vi "Create All Message Queues.vi"(8 "error in (no error)":errorcluster) -> (0 "error out":errorcluster, 3 "Message Queues out":T1)   [LabVIEW 2026, in "Temp Monitor Message Queue.lvlib"]
doc: "This VI creates and initializes all the message queues for the Temperature Monitoring application."
uses:
  Temp Monitor Message Queue.lvlib
  All Message Queues.ctl
  Message Cluster.ctl
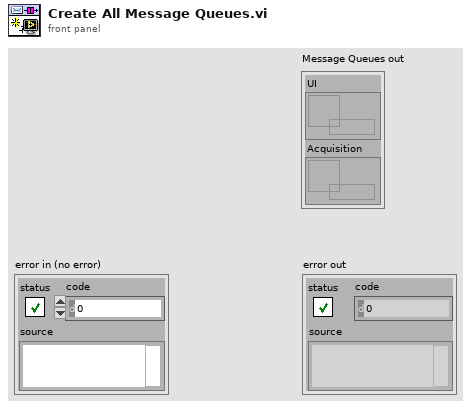
[diagram p1: front panel]
types:
  T1 = typedef "Temp Monitor Message Queue.lvlib/All Message Queues.ctl" = cluster{"UI":refnum<queue>, "Acquisition":refnum<queue>}
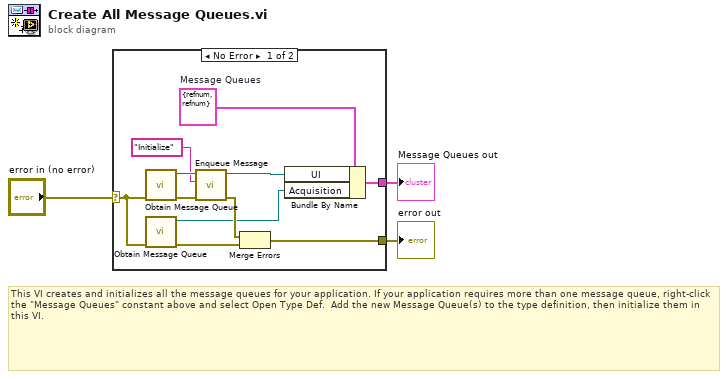
[diagram p0: block diagram]
diagram:
  # "This VI creates and initializes all the message queues for your application. If your application requires more than one message queue, right-click the \"Message Queues\" constant above and select Open Type Def.  Add the new Message Queue(s) to the type definition, then initialize them in this VI."
  n1 = case shown="No Error" "error in (no error)" {
    selector: "error in (no error)" -> [w9 w15]
    tunnel: [w6 w15] -> w3
    tunnel: [w12 _] -> w2
    frame No Error {
      w13 = T1 {"UI"=refnum, "Acquisition"=refnum}  # Message Queues
      n2 = call "Obtain Message Queue.vi"("error in (no error)"=w9) -> ("error out"=w11:errorcluster, "Message Queue"=w10:refnum<queue>)  [unwired: 9 in]
      n3 = call "Obtain Message Queue.vi"("error in (no error)"=w9) -> ("error out"=w4:errorcluster, "Message Queue"=w5:refnum<queue>)  [unwired: 9 in]
      n4 = call "Enqueue Message.vi"("error in (no error)"=w11, "Message"="Initialize", "Message Queue"=w10) -> ("error out"=w14:errorcluster, "dup Message Queue"=w7:refnum<queue>)  [unwired: 7 in]
      n5 = Merge Errors(w14, w4) -> (w6:errorcluster)
      n6 = Bundle By Name(cluster=w13, "UI"=w7, "Acquisition"=w5) -> (w12:T1)
    }
    frame Error {
    }
  }
  "Message Queues out" <- w2
  "error out" <- w3
